vi "Format Error Terminals.vi"(8 "error in (no error)":errorcluster, 11 "vi path":path) -> (0 "error out":errorcluster)   [LabVIEW 2023]
uses:
  <vilib>/Utility/traverseref.llb/VI Scripting - Traverse.lvlib
  <vilib>/Utility/traverseref.llb/TRef TravTarget.ctl
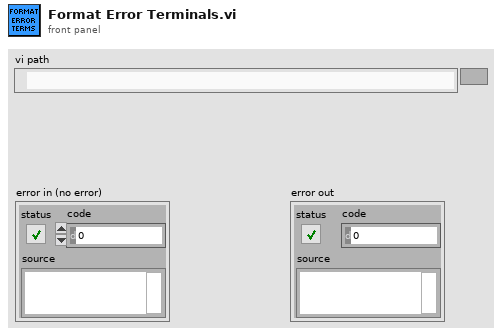
[diagram p1: front panel]
types:
  T1 = typedef "TRef TravTarget.ctl" = enum16{"FP", "BD", "Other"}
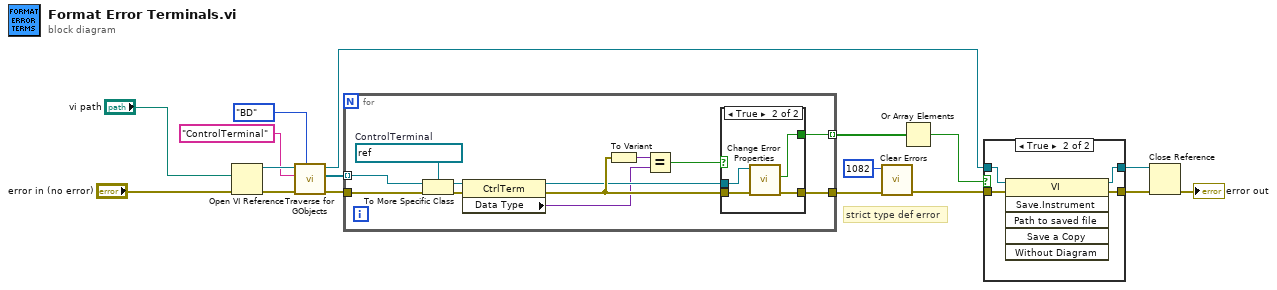
[diagram p0: block diagram]
diagram:
  # "strict type def error"
  n1 = Open VI Reference(vi path="vi path", error in (no error)="error in (no error)") -> (vi reference=w11:refnum<vi>, error out=w12:errorcluster)  [unwired: 4 in]
  n2 = call <vilib>:"Traverse for GObjects.vi"("Traverse Target"=TRef_TravTarget."BD", "error in (no error)"=w12, "Class Name"="ControlTerminal", "VI Refnum"=w11) -> ("error out"=w9:errorcluster, "References"=w8:refnum<vi>[], "dup VI Refnum"=w2:refnum<vi>)  [unwired: 4 in, 1 out]
  n3 = for {
    tunnel: w8 -> [w29] mode=indexing
    tunnel: [w18] -> w3 mode=indexing
    tunnel: w9 -> [w25]
    tunnel: [w21] -> w5
    w28 = refnum<vi> refnum  # ControlTerminal
    n4 = To More Specific Class(target class=w28, reference=w29, error in=w25) -> (specific class reference=w27:refnum<vi>, error out=w26:errorcluster)
    n5 = property class="CtrlTerm"(reference=w27, error in=w26) -> (reference out=w20:refnum<vi>, error out=w23:errorcluster, "Data Type"=w19:variant)
    n6 = To Variant(anything=w23) -> (Variant=w24:variant)
    n7 = Equal?(x=w24, y=w19) -> (x = y?=w22:bool)
    n8 = case shown="True" w22 {
      tunnel: w23 -> [w30 w34]
      tunnel: [w30 w33] -> w21
      tunnel: w20 -> [_ w32]
      tunnel: [_ w31] -> w18
      frame False {
      }
      frame True {
        n9 = call "Change Error Properties.vi"("error in (no error)"=w34, "CtrlTerm Ref"=w32) -> ("error out"=w33:errorcluster, "Changed?"=w31:bool)  [unwired: 8 in]
      }
    }
  }
  n10 = call <vilib>:"Clear Errors.vi"("error in (no error)"=w5, "specific error code to clear (0: all)"=1082) -> ("error out"=w1:errorcluster)  [unwired: 4 in, 1 out]
  n11 = Or Array Elements(Boolean array=w3) -> (logical OR=w6:bool)
  n12 = case shown="True" w6 {
    tunnel: w1 -> [w36 w40]
    tunnel: [w36 w39] -> w14
    tunnel: [w35 w38] -> w13
    tunnel: w2 -> [w35 w37]
    frame False {
    }
    frame True {
      n13 = invoke class="VI" method="Save.Instrument"(reference=w37, error in=w40) -> (reference out=w38:refnum<vi>, error out=w39:errorcluster)  [unwired: 4 in, 4 out]
    }
  }
  n14 = Close Reference(reference=w13, error in (no error)=w14) -> (error out=→"error out":errorcluster)
